vi "Initialize Actor.vi"(7 "Host Name":string, 8 "error in (no error)":errorcluster, 9 "Actor Name":string, 10 "Message Broker Interface":refnum<class "Message Broker Interface.lvclass">, 11 "Car Wash eStop in":refnum<class "Car Wash eStop.lvclass">) -> (0 "error out":errorcluster, 3 "Car Wash eStop out":refnum<class "Car Wash eStop.lvclass">)   [LabVIEW 2016, in "CLD Exam - Car Wash.lvlib" / "Car Wash eStop.lvclass"]
doc: "--\nCopyright © 2017 Composed SystemsI All rights reserved.\n\nAuthor: Jon McBee <jon.mcbee@composed.io>\n\nThis library is provided \"AS IS\" ,WITHOUT WARRANTIES OR\nCONDITIONS OF ANY KIND, either express or implied.\n\nComposed Systems -- composed.io\n\nStream 0.0.1.1\nJon McBee - Composed Systems\nCopyright (c) 2017, Composed Systems"
uses:
  Car Wash eStop.lvclass
  Mediator/Classes/Message Broker Interface/Message Broker Interface.lvclass
  Mediator/Classes/Mediated Synchronous Actor/Mediated Synchronous Actor.lvclass
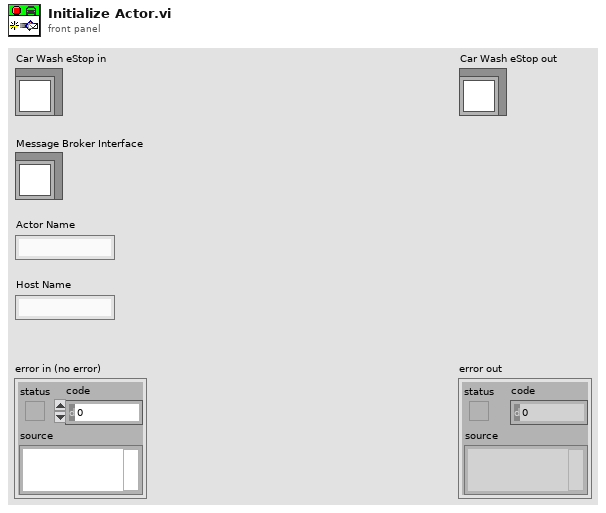
[diagram p1: front panel]
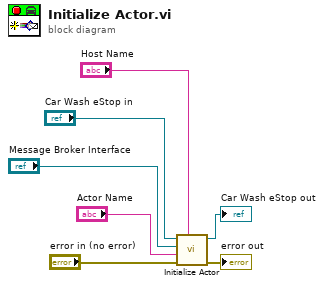
[diagram p0: block diagram]
diagram:
  n1 = call-parent "Initialize Actor.vi"("Host Name"="Host Name", "error in (no error)"="error in (no error)", "Actor Name"="Actor Name", "Message Broker Interface"="Message Broker Interface", "Mediated Synchronous Actor in"="Car Wash eStop in") -> ("error out"=→"error out":errorcluster, "Mediated Synchronous Actor out"=→"Car Wash eStop out":refnum<class "Car Wash eStop.lvclass">)  [unwired: 5 in]
